vi "PruebaCounter.vi"() -> ()   [LabVIEW 2014, in "MSX-E3711_dll.lvlib"]
uses:
  MSX-E3711_dll.lvlib
  Typedef/Config Data.ctl
  Typedef/Connection Data.ctl
  E:/Repositorio Magnis/INF002/v0/Modules/HAL/Drivers/Sync/ADDI-DATA MSX-E3711/API/MSXE371x.dll
  MSXE371x.dll
  E:/Repositorio Magnis/INF002/v0/Modules/HAL/Drivers/Sync/ADDI-DATA MSX-E3711/API/MXCommon.dll
  MXCommon.dll
panel:
  in  "IncCounter":T1
  in  "Counter Clear":bool
  out "CounterValue":u64
  in  "error in (no error)":errorcluster
  out "error out":errorcluster
  in  "stop":bool
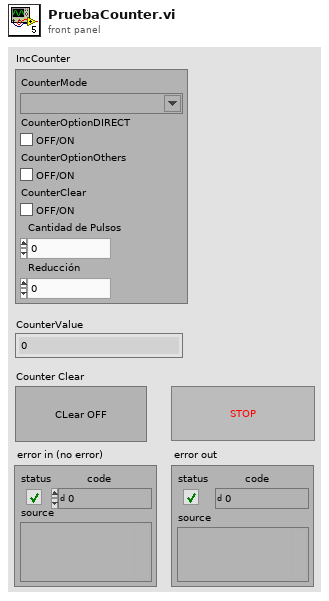
[diagram p1: front panel]
types:
  T1 = cluster{"CounterMode":string, "CounterOptionDIRECT  ":bool, "CounterOptionOthers":bool, "CounterClear ":bool, "Cantidad de Pulsos":sgl, "Reducción":sgl}
  T2 = typedef "MSX-E3711_dll.lvlib/Connection Data.ctl" = cluster{"MX371x refnum":refnum<k24>, "IP":string, "Connection ID ":refnum<k5>, "MXCommon refnum":refnum<k24>}
  T3 = typedef "MSX-E3711_dll.lvlib/Config Data.ctl" = cluster{"Auto Refresh":cluster{"Average Mode":u64, "Average Value":u64, "Trigger Mask":u64, "Trigger Mode":u64, "Hardware Trigger Edge":u64, "Hardware Trigger Count":u64, "By Trigger Nbr Of Seq To Acquire":u64, "Time stamp":bool, "Analog Output(mm)":bool, "Invert value":bool, "Temperature value":bool, "Incremental counter value":bool, "Diff. mode":bool}, "Gain":sgl[], "Offset":sgl[], "Index":u64, "Range":sgl, "Sequence":cluster{"Nbr Of Sequence":u64, "Nbr Max Sequence To Transfer":u64, "Delay Mode":u64, "Delay Time Unit":u64, "Delay Value":u64, "Trigger Mask":u64, "Trigger Mode":u64, "Hardware Trigger Edge":u64, "Hardware Trigger Count":u64, "By Trigger Nbr Of Seq To Acquire":u64, "Time stamp":bool, "Sequence counter information":bool, "Analog Output(mm)":bool, "Invert value":bool, "Temperature value":bool, "Incremental counter value":bool, "Diff. mode":bool}, "Enable DIO":bool, "IncCounter":cluster{"CounterMode":string, "CounterOptionDIRECT  ":bool, "CounterOptionOthers":bool, "CounterClear ":bool, "Cantidad de Pulsos":sgl, "Reducción":sgl}, "IncTemperature":cluster{"ConnectedTempSensor":string, "ConvertMode":string, "InitGainSelection":string, "FrequencySelection":string, "PowerSaveMode":bool, "GainSelection":string, "RefValue":dbl}}
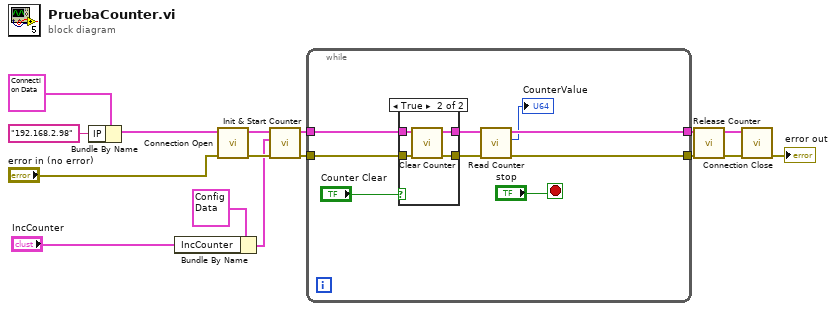
[diagram p0: block diagram]
diagram:
  w5 = T2 {"MX371x refnum"=refnum, "IP"="192.168.2.98", "Connection ID "=refnum, "MXCommon refnum"=refnum} ("Connection Data In")
  n1 = Bundle By Name(cluster=w5, "IP"="192.168.2.98") -> ()  [unwired: 1 out]
  n2 = Bundle By Name(cluster=T3 {"Auto Refresh"={"Average Mode"=0, "Average Value"=0, "Trigger Mask"=0, "Trigger Mode"=0, "Hardware Trigger Edge"=0, "Hardware Trigger Count"=0, "By Trigger Nbr Of Seq To Acquire"=0, "Time stamp"=FALSE, "Analog Output(mm)"=FALSE, "Invert value"=FALSE, "Temperature value"=FALSE, "Incremental counter value"=FALSE, "Diff. mode"=FALSE}, "Gain"=[], "Offset"=[], "Index"=0, "Range"=0.0, "Sequence"={"Nbr Of Sequence"=0, "Nbr Max Sequence To Transfer"=800, "Delay Mode"=0, "Delay Time Unit"=0, "Delay Value"=0, "Trigger Mask"=5, "Trigger Mode"=0, "Hardware Trigger Edge"=0, "Hardware Trigger Count"=0, "By Trigger Nbr Of Seq To Acquire"=1, "Time stamp"=FALSE, "Sequence counter information"=TRUE, "Analog Output(mm)"=FALSE, "Invert value"=FALSE, "Temperature value"=FALSE, "Incremental counter value"=FALSE, "Diff. mode"=FALSE}, "Enable DIO"=FALSE, "IncCounter"={"CounterMode"="1", "CounterOptionDIRECT  "=FALSE, "CounterOptionOthers"=FALSE, "CounterClear "=FALSE, "Cantidad de Pulsos"=0.0, "Reducción"=0.0}, "IncTemperature"={"ConnectedTempSensor"="", "ConvertMode"="", "InitGainSelection"="", "FrequencySelection"="", "PowerSaveMode"=FALSE, "GainSelection"="", "RefValue"=0.0}} ("Config Data"), "IncCounter"="IncCounter") -> (w2:T3)
  n3 = call "Connection Open.vi"("error in (no error)"="error in (no error)", "Connection Data In"=w5) -> ("error out"=w14:errorcluster, "Connection Data Out"=w15:T2)  [unwired: 8 in]
  n4 = call "Init & Start Counter.vi"("error in (no error)"=w14, "Config Data"=w2, "Connection Data In"=w15) -> ("error out"=w13:errorcluster, "Connection Data Out"=w12:T2)  [unwired: 7 in]
  n5 = while {
    tunnel: w13 -> [w20]
    tunnel: w12 -> [w21]
    tunnel: [w22] -> w7
    tunnel: [w23] -> w6
    stop <- "stop" stop-if-true
    n6 = case shown="True" "Counter Clear" {
      tunnel: w21 -> [w26 w30]
      tunnel: w20 -> [w25 w28]
      tunnel: [w26 w29] -> w18
      tunnel: [w25 w27] -> w17
      frame False {
      }
      frame True {
        n7 = call "Clear Counter.vi"("error in (no error)"=w28, "Connection Data In"=w30) -> ("error out"=w27:errorcluster, "Connection Data Out"=w29:T2)  [unwired: 8 in]
      }
    }
    n8 = call "Read Counter.vi"("error in (no error)"=w17, "Connection Data In"=w18) -> ("error out"=w22:errorcluster, "CounterValue"=→"CounterValue":u64, "Connection Data Out"=w23:T2)  [unwired: 7 in]
  }
  n9 = call "Release Counter.vi"("error in (no error)"=w7, "Connection Data In"=w6) -> ("error out"=w8:errorcluster, "Connection Data Out"=w9:T2)  [unwired: 8 in]
  n10 = call "Connection Close.vi"("error in (no error)"=w8, "Connection Data In"=w9) -> ("error out"=→"error out":errorcluster)  [unwired: 8 in, 1 out]
